vi "h.COMM.Close Connection.vi"(8 "error in":errorcluster, 11 "Connection ID":refnum<k5>) -> (0 "error out":errorcluster)   [LabVIEW 2016, in "h.Library.lvlib"]
doc: "Closes a previously opened socket connection to a Hyperion instrument."
uses:
  h.Library.lvlib
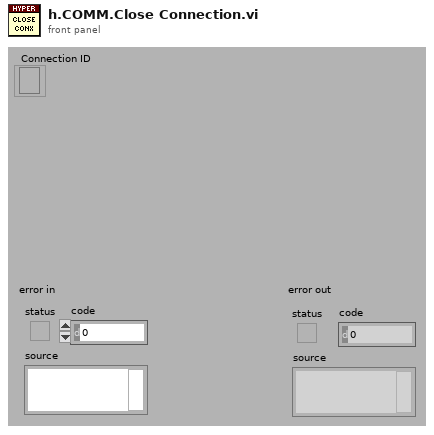
[diagram p1: front panel]
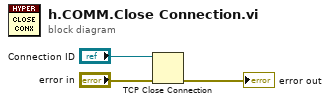
[diagram p0: block diagram]
diagram:
  n1 = TCP Close Connection(connection ID="Connection ID", error in (no error)="error in") -> (error out=→"error out":errorcluster)  [unwired: 1 in, 1 out]
